vi "Read Name.vi"(8 "error in (no error)":errorcluster, 11 "Endpoint":refnum<class "Endpoint.lvclass">) -> (0 "error out":errorcluster, 2 "Name":string, 3 "Endpoint out":refnum<class "Endpoint.lvclass">)   [LabVIEW 2015, in "NI_AWS_SNS.lvlib" / "Endpoint.lvclass"]
uses:
  Endpoint.lvclass
  Core/ARN/ARN.lvclass
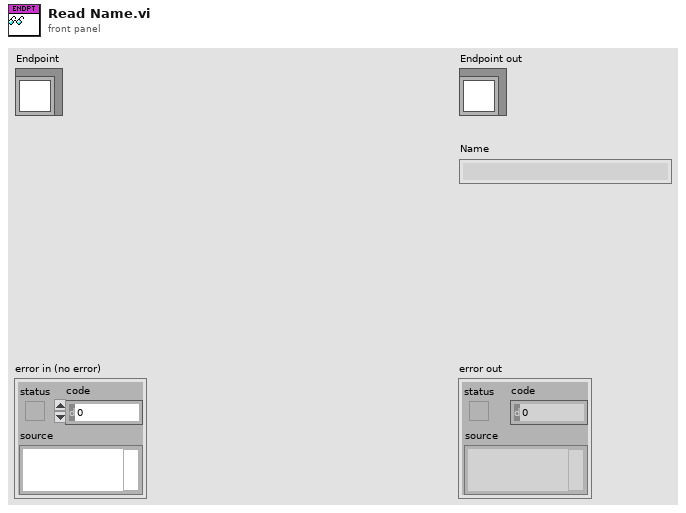
[diagram p1: front panel]
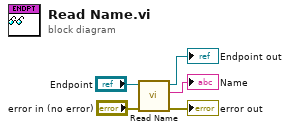
[diagram p0: block diagram]
diagram:
  n1 = call-parent "Read Name.vi"("error in (no error)"="error in (no error)", "ARN"="Endpoint") -> ("error out"=→"error out":errorcluster, "Name"=→"Name":string, "ARN out"=→"Endpoint out":refnum<class "Endpoint.lvclass">)  [unwired: 7 in]
